vi "Validate Experiment Location.vi"(11 "Experiment Location":path) -> (2 "Error (if invalid)":string, 3 "Valid Experiment Directory?":bool)   [LabVIEW 2020, in "Experiment Manager.lvlib"]
uses:
  Experiment Manager.lvlib
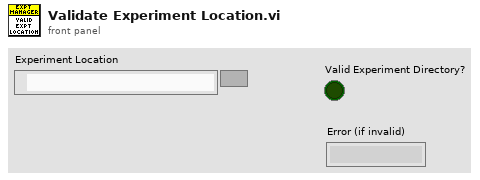
[diagram p1: front panel]
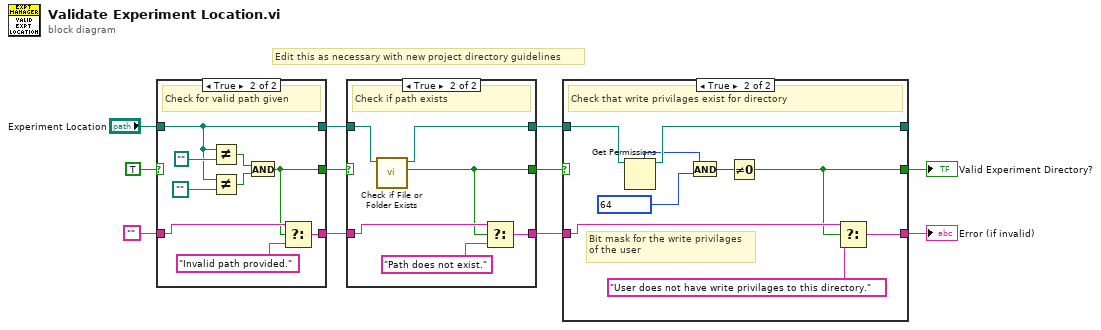
[diagram p0: block diagram]
diagram:
  # "Edit this as necessary with new project directory guidelines"
  n1 = case shown="True" TRUE {
    selector: TRUE -> [w13 _]
    tunnel: [w14 w19] -> w8
    tunnel: "Experiment Location" -> [w14 w19]
    tunnel: [w13 w17] -> w7
    tunnel: [w12 w15] -> w3
    tunnel: "" -> [w12 w18]
    frame False {
    }
    frame True {
      # "Check for valid path given"
      n2 = Not Equal?(x=w19, y=path "") -> (x != y?=w23:bool)
      n3 = Not Equal?(x=w19, y=path "") -> (x != y?=w22:bool)
      n4 = And(x=w23, y=w22) -> (x .and. y?=w17:bool)
      n5 = Select(t=w18, s=w17, f="Invalid path provided.") -> (s? t:f=w15:string)
    }
  }
  n6 = case shown="True" w7 {
    selector: w7 -> [w25 _]
    tunnel: [w26 w32] -> w11
    tunnel: w8 -> [w26 w31]
    tunnel: [w25 w28] -> w10
    tunnel: [w24 w30] -> w2
    tunnel: w3 -> [w24 w29]
    frame False {
    }
    frame True {
      # "Check if path exists"
      n7 = call <vilib>:"Check if File or Folder Exists.vi"("path"=w31) -> ("file or folder exists?"=w28:bool, "dup path"=w32:path)  [unwired: 8 in, 1 out]
      n8 = Select(t=w29, s=w28, f="Path does not exist.") -> (s? t:f=w30:string)
    }
  }
  n9 = case shown="True" w10 {
    selector: w10 -> [w34 _]
    tunnel: [w35 w43] -> _
    tunnel: w11 -> [w35 w44]
    tunnel: [w34 w37] -> w9
    tunnel: [w33 w38] -> w1
    tunnel: w2 -> [w33 w39]
    frame False {
    }
    frame True {
      # "Bit mask for the write privilages\nof the user"
      # "Check that write privilages exist for directory"
      n10 = Get Permissions(11:w44) -> (3:w43:path, 5:w41:i16)  [unwired: 1 in, 3 out]
      n11 = And(x=w41, y=u16 64) -> (x .and. y?=w40:u16)
      n12 = Not Equal To 0?(x=w40) -> (x != 0?=w37:bool)
      n13 = Select(t=w39, s=w37, f="User does not have write privilages to this directory.") -> (s? t:f=w38:string)
    }
  }
  "Valid Experiment Directory?" <- w9
  "Error (if invalid)" <- w1
